vi "BatchProcess_AllFile.vi"() -> ()   [LabVIEW 2015, in "EMG.lvclass"]
uses:
  EMG.lvclass
panel:
  in  "stop":bool
  in  "Functions":enum16{"Reduce File Size", "Change Mod Date"}(ring)
  in  "File Pattern":string="*.txt"
  out "Current File":string
  out "Current File":i32
  out "Total Files":i32
  in  "Parent Folder of subject folder":path
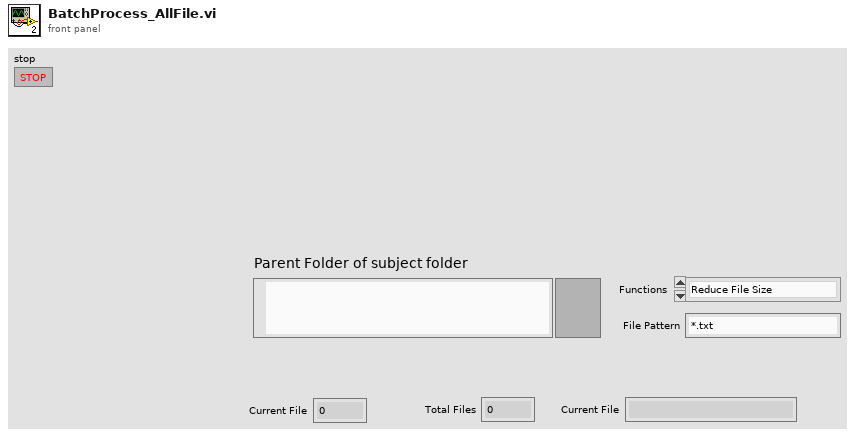
[diagram p1: front panel]
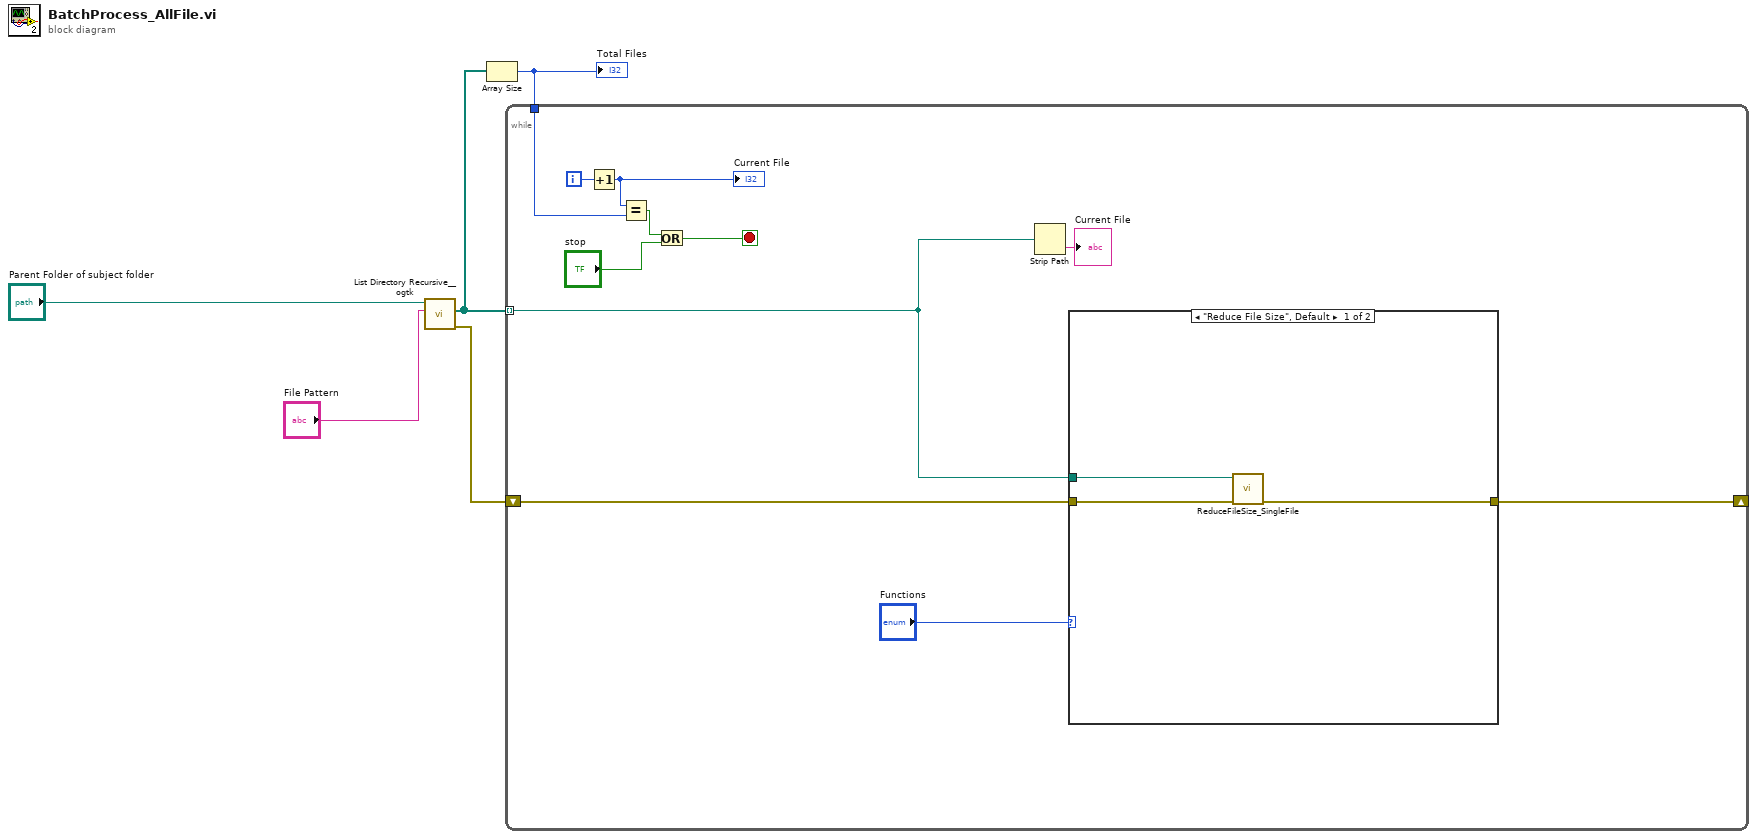
[diagram p0: block diagram]
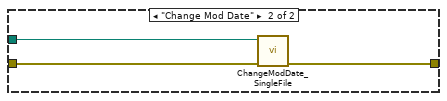
[diagram p2: hidden frame]
diagram:
  n1 = call <userlib>:"List Directory Recursive__ogtk.vi"("pattern"="File Pattern", "Path"="Parent Folder of subject folder") -> ("error out"=w5:errorcluster, "file paths"=w2:path[])  [unwired: 6 in, 2 out]
  n2 = Array Size(array=w2) -> (size(s)=w1:i32)
  "Total Files" <- w1
  n3 = while {
    tunnel: w2 -> [w12] mode=indexing
    shift-right: [w15] -> _
    shift-left: w5 -> [w16]
    tunnel: w1 -> [w8]
    i -> [w7]
    stop <- w11 stop-if-true
    n4 = Increment(x=w7) -> (x+1=w6:i32)
    "Current File" <- w6
    n5 = Equal?(x=w6, y=w8) -> (x = y?=w9:bool)
    n6 = Or(x=w9, y="stop") -> (x .or. y?=w11:bool)
    n7 = Strip Path(path=w12) -> (name=→"Current File":string)  [unwired: 1 out]
    n8 = case shown="\"Reduce File Size\", Default" "Functions" {
      tunnel: w16 -> [w19 w22]
      tunnel: [w18 w20] -> w15
      tunnel: w12 -> [w17 w21]
      frame "Reduce File Size", Default {
        n9 = call "ReduceFileSize_SingleFile.vi"("error in (no error)"=w19, "appended path"=w17) -> ("error out"=w18:errorcluster)  [unwired: 8 in, 1 out]
      }
      frame "Change Mod Date" {
        n10 = call "ChangeModDate_SingleFile.vi"("error in (no error)"=w22, "appended path"=w21) -> ("error out"=w20:errorcluster)  [unwired: 7 in, 2 out]
      }
    }
  }
